vi "SaveConfig.vi"(8 "error in (no error)":errorcluster, 9 "Cluster":T1 {"Screw 8" items=["0", "1", "2", "3", "4", "5", "6", "7", "8", "9", "10"]; "Screw 7" items=["0", "1", "2", "3", "4", "5", "6", "7", "8", "9", "10"]; "Screw 6" items=["0", "1", "2", "3", "4", "5", "6", "7", "8", "9", "10"]; "Screw 5" items=["0", "1", "2", "3", "4", "5", "6", "7", "8", "9", "10"]; "Screw 4" items=["0", "1", "2", "3", "4", "5", "6", "7", "8", "9", "10"]; "Screw 3" items=["0", "1", "2", "3", "4", "5", "6", "7", "8", "9", "10"]; "Screw 2" items=["0", "1", "2", "3", "4", "5", "6", "7", "8", "9", "10"]; "M6_Camera" items=["0", "1", "2", "3", "4", "5", "6", "7", "8", "9", "10", "11", "12", "13", "14", "15", "16", "17", "18", "19", "20"]; "L/R" items=["NA", "RHD-VAC", "RHD-HVAC", "LHD-VAC", "LHD-HVAC", ""]}, 10 "PN":string, 11 "Path":string) -> (0 "error out":errorcluster)   [LabVIEW 2020]
uses:
  NewPNConfig.ctl
  <vilib>/Utility/config.llb/Write Key (String).vi
  <vilib>/Utility/config.llb/Write Key (U32).vi
  <vilib>/Utility/config.llb/NI_LVConfig.lvlib
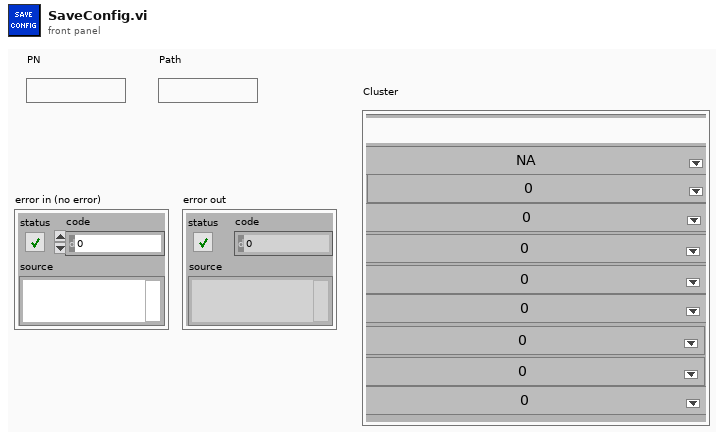
[diagram p1: front panel]
types:
  T1 = typedef "NewPNConfig.ctl" = cluster{"L/R":u8, "PN":string, "M6_Camera":u16, "Screw 2":u16, "Screw 3":u16, "Screw 4":u16, "Screw 5":u16, "Screw 6":u16, "Screw 7":u16, "Screw 8":u16}
  T2 = typedef "NI_LVConfig.lvlib/Config Data RefNum.ctl" = refnum<k1>
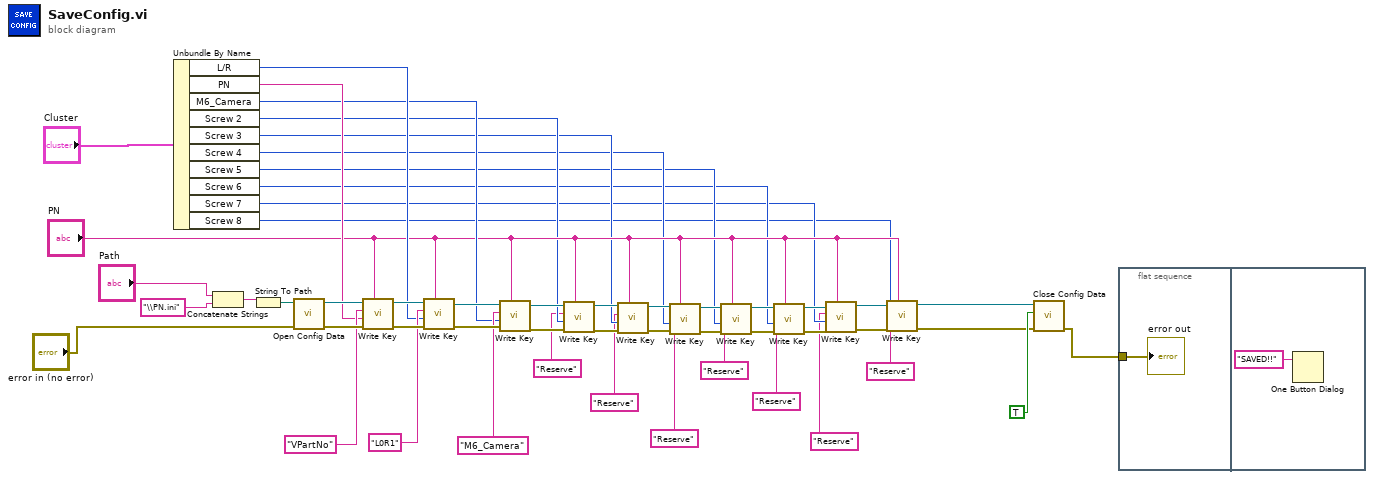
[diagram p0: block diagram]
diagram:
  n1 = Unbundle By Name("Cluster") -> ("L/R"=w33:u8, "PN"=w34:string, "M6_Camera"=w32:u16, "Screw 2"=w14:u16, "Screw 3"=w13:u16, "Screw 4"=w12:u16, "Screw 5"=w11:u16, "Screw 6"=w10:u16, "Screw 7"=w9:u16, "Screw 8"=w8:u16)
  n2 = Concatenate Strings("Path", "\\PN.ini") -> (w47:string)
  n3 = String To Path(string=w47) -> (path=w49:path)
  n4 = call <vilib>:"Open Config Data.vi"("error in (no error)"="error in (no error)", "configuration file path"=w49) -> ("error out"=w44:errorcluster, "refnum"=w38:T2)  [unwired: 7 in, 1 out]
  n5 = call-poly <vilib>:"Write Key.vi"("section"="PN", "error in (no error)"=w44, "value"=w34, "key"="VPartNo", "refnum"=w38) -> ("error out"=w43:errorcluster, "refnum out"=w39:T2)  [unwired: 4 in, 1 out]
  n6 = call-poly <vilib>:"Write Key.vi"("section"="PN", "error in (no error)"=w43, "value"=w33, "key"="L0R1", "refnum"=w39) -> ("error out"=w42:errorcluster, "refnum out"=w40:T2)  [unwired: 4 in, 1 out]
  n7 = call-poly <vilib>:"Write Key.vi"("section"="PN", "error in (no error)"=w42, "value"=w32, "key"="M6_Camera", "refnum"=w40) -> ("error out"=w31:errorcluster, "refnum out"=w23:T2)  [unwired: 4 in, 1 out]
  n8 = call-poly <vilib>:"Write Key.vi"("section"="PN", "error in (no error)"=w31, "value"=w14, "key"="Reserve", "refnum"=w23) -> ("error out"=w29:errorcluster, "refnum out"=w22:T2)  [unwired: 4 in, 1 out]
  n9 = call-poly <vilib>:"Write Key.vi"("section"="PN", "error in (no error)"=w29, "value"=w13, "key"="Reserve", "refnum"=w22) -> ("error out"=w30:errorcluster, "refnum out"=w21:T2)  [unwired: 4 in, 1 out]
  n10 = call-poly <vilib>:"Write Key.vi"("section"="PN", "error in (no error)"=w30, "value"=w12, "key"="Reserve", "refnum"=w21) -> ("error out"=w28:errorcluster, "refnum out"=w20:T2)  [unwired: 4 in, 1 out]
  n11 = call-poly <vilib>:"Write Key.vi"("section"="PN", "error in (no error)"=w28, "value"=w11, "key"="Reserve", "refnum"=w20) -> ("error out"=w27:errorcluster, "refnum out"=w19:T2)  [unwired: 4 in, 1 out]
  n12 = call-poly <vilib>:"Write Key.vi"("section"="PN", "error in (no error)"=w27, "value"=w10, "key"="Reserve", "refnum"=w19) -> ("error out"=w26:errorcluster, "refnum out"=w18:T2)  [unwired: 4 in, 1 out]
  n13 = call-poly <vilib>:"Write Key.vi"("section"="PN", "error in (no error)"=w26, "value"=w9, "key"="Reserve", "refnum"=w18) -> ("error out"=w25:errorcluster, "refnum out"=w17:T2)  [unwired: 4 in, 1 out]
  n14 = call-poly <vilib>:"Write Key.vi"("section"="PN", "error in (no error)"=w25, "value"=w8, "key"="Reserve", "refnum"=w17) -> ("error out"=w24:errorcluster, "refnum out"=w16:T2)  [unwired: 4 in, 1 out]
  n15 = call <vilib>:"Close Config Data.vi"("error in (no error)"=w24, "write file if changed (T)"=TRUE, "refnum"=w16) -> ("error out"=w41:errorcluster)  [unwired: 7 in, 1 out]
  n16 = flat-sequence {
    tunnel: w41 -> [w52]
    frame #0 {
      "error out" <- w52
    }
    frame #1 {
      n17 = One Button Dialog(message="SAVED!!") -> ()  [unwired: 1 in, 1 out]
    }
  }
